vi "quadraticEq.vi"(1 "each_char":string) -> (2 "String":string)   [LabVIEW 2018]
panel:
  out "Def":string
  out "c":string
  out "b":string
  out "a":string
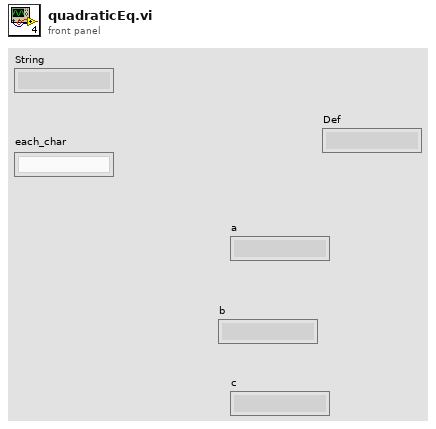
[diagram p1: front panel]
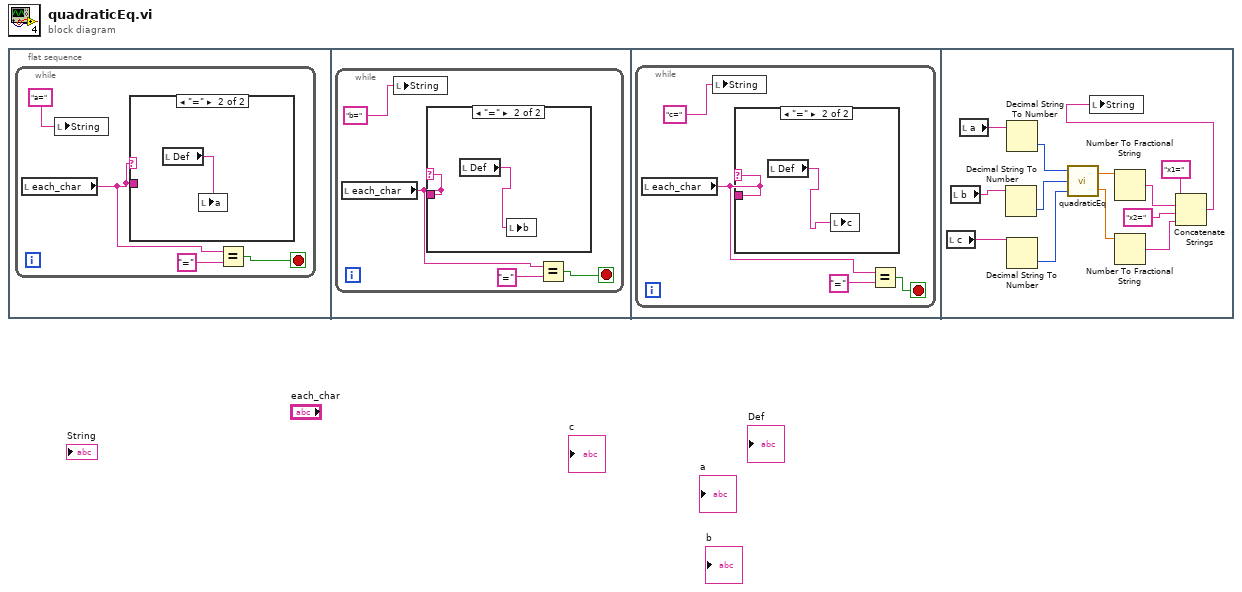
[diagram p0: block diagram]
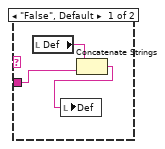
[diagram p2: hidden frame]
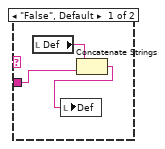
[diagram p3: hidden frame]
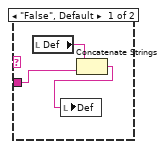
[diagram p4: hidden frame]
diagram:
  n1 = flat-sequence {
    frame #0 {
      n2 = while {
        stop <- w2 stop-if-true
        n3 = local read "each_char"() -> (w3:string)
        n4 = local write "String"("a=" ("String")) -> ()
        n5 = case shown="\"=\"" w3 {
          tunnel: w3 -> [w7 _]
          frame "False", Default {
            n6 = local read "Def"() -> (w6:string)
            n7 = Concatenate Strings(w6, w7) -> (w5:string)
            n8 = local write "Def"(w5) -> ()
          }
          frame "=" {
            n9 = local read "Def"() -> (w8:string)
            n10 = local write "a"(w8) -> ()
          }
        }
        n11 = Equal?(x=w3, y="=") -> (x = y?=w2:bool)
      }
    }
    frame #1 {
      n12 = while {
        stop <- w9 stop-if-true
        n13 = local read "each_char"() -> (w11:string)
        n14 = local write "String"("b=" ("String")) -> ()
        n15 = case shown="\"=\"" w11 {
          tunnel: w11 -> [w15 _]
          frame "False", Default {
            n16 = local read "Def"() -> (w14:string)
            n17 = Concatenate Strings(w14, w15) -> (w13:string)
            n18 = local write "Def"(w13) -> ()
          }
          frame "=" {
            n19 = local read "Def"() -> (w16:string)
            n20 = local write "b"(w16) -> ()
          }
        }
        n21 = Equal?(x=w11, y="=") -> (x = y?=w9:bool)
      }
    }
    frame #2 {
      n22 = while {
        stop <- w17 stop-if-true
        n23 = local read "each_char"() -> (w19:string)
        n24 = local write "String"("c=" ("String")) -> ()
        n25 = case shown="\"=\"" w19 {
          tunnel: w19 -> [w23 _]
          frame "False", Default {
            n26 = local read "Def"() -> (w22:string)
            n27 = Concatenate Strings(w22, w23) -> (w21:string)
            n28 = local write "Def"(w21) -> ()
          }
          frame "=" {
            n29 = local read "Def"() -> (w24:string)
            n30 = local write "c"(w24) -> ()
          }
        }
        n31 = Equal?(x=w19, y="=") -> (x = y?=w17:bool)
      }
    }
    frame #3 {
      n32 = local read "c"() -> (w33:string)
      n33 = local read "b"() -> (w35:string)
      n34 = local read "a"() -> (w37:string)
      n35 = Decimal String To Number(string=w35) -> (number=w34:i32)  [unwired: 2 in, 1 out]
      n36 = Decimal String To Number(string=w37) -> (number=w36:i32)  [unwired: 2 in, 1 out]
      n37 = Decimal String To Number(string=w33) -> (number=w32:i32)  [unwired: 2 in, 1 out]
      n38 = call "quadraticEq.vi"("c"=w32, "b"=w34, "a"=w36) -> ("x2"=w28:dbl, "x1"=w31:dbl)
      n39 = Number To Fractional String(number=w31) -> (F-format string=w30:string)  [unwired: 3 in]
      n40 = Number To Fractional String(number=w28) -> (F-format string=w26:string)  [unwired: 3 in]
      n41 = Concatenate Strings("x1=" ("string"), w30, "x2=" ("string"), w26) -> (w25:string)
      n42 = local write "String"(w25) -> ()
    }
  }
